vi "Contour.vi"(8 "error in (no error)":errorcluster, 10 "ContourParameter":T3={"ROI"={"Global Rectangle"=[], "Contours"=[]}, "Search Direction"=enum."Rect Left To Right", "Curve Extraction"={"Extraction Mode"=0, "Edge Threshold"=75, "Edge Filter Size"=1, "Min Length"=25, "Search Step Size"=15, "Max Endpoint Gap"=10, "Subpixel"=TRUE}, "Contour Selection"=enum."Closest To Search Start", "Curve Connection"=[]} {"Curve Connection"."Max" format="%.2f"; "Curve Connection"."Min" format="%.2f"; "Curve Connection"."Match Constraints" items=["Distance (pixel)", "Angle Difference (degrees)", "Connectivity Distance (pixel)", "Gradient Difference (degrees)"]; "Curve Extraction"."Extraction Mode" items=["Normal", "Uniform Regions"]; "Curve Extraction"."Edge Filter Size" items=["Fine", "Normal", "Contour Tracing"]; "Curve Extraction"."Max Endpoint Gap" min=0; "Curve Extraction"."Search Step Size" min=1 max=255 step=1; "Curve Extraction"."Min Length" min=0; "Curve Extraction"."Edge Threshold" min=1 max=350 step=1; "ROI"."Contours"."Type" items=["No Selection", "Point", "Line", "Rectangle", "Oval", "Polygon", "Free", "Annulus", "Unused2", "Unused3", "Broken Line", "Free Hand Line", "Rotated Rectangle"]}, 11 "Image In":T2) -> (0 "error out":errorcluster, 2 "ContourResult":T1, 3 "Image Out":T2)   [LabVIEW 2019]
uses:
  <vilib>/vision/Image Controls.llb/IMAQ Image.ctl
  Controls/Contour/Analysis_Contour_Parameter.ctl
  <vilib>/vision/Contour.llb/IMAQ Contour Curve Extraction.ctl
  <vilib>/vision/Contour.llb/IMAQ Connect Range Setting.ctl
  Controls/Contour/Analysis_Contour_Result.ctl
  <vilib>/vision/NI_Vision_Development_Module.lvlib
panel:
  # "Range"
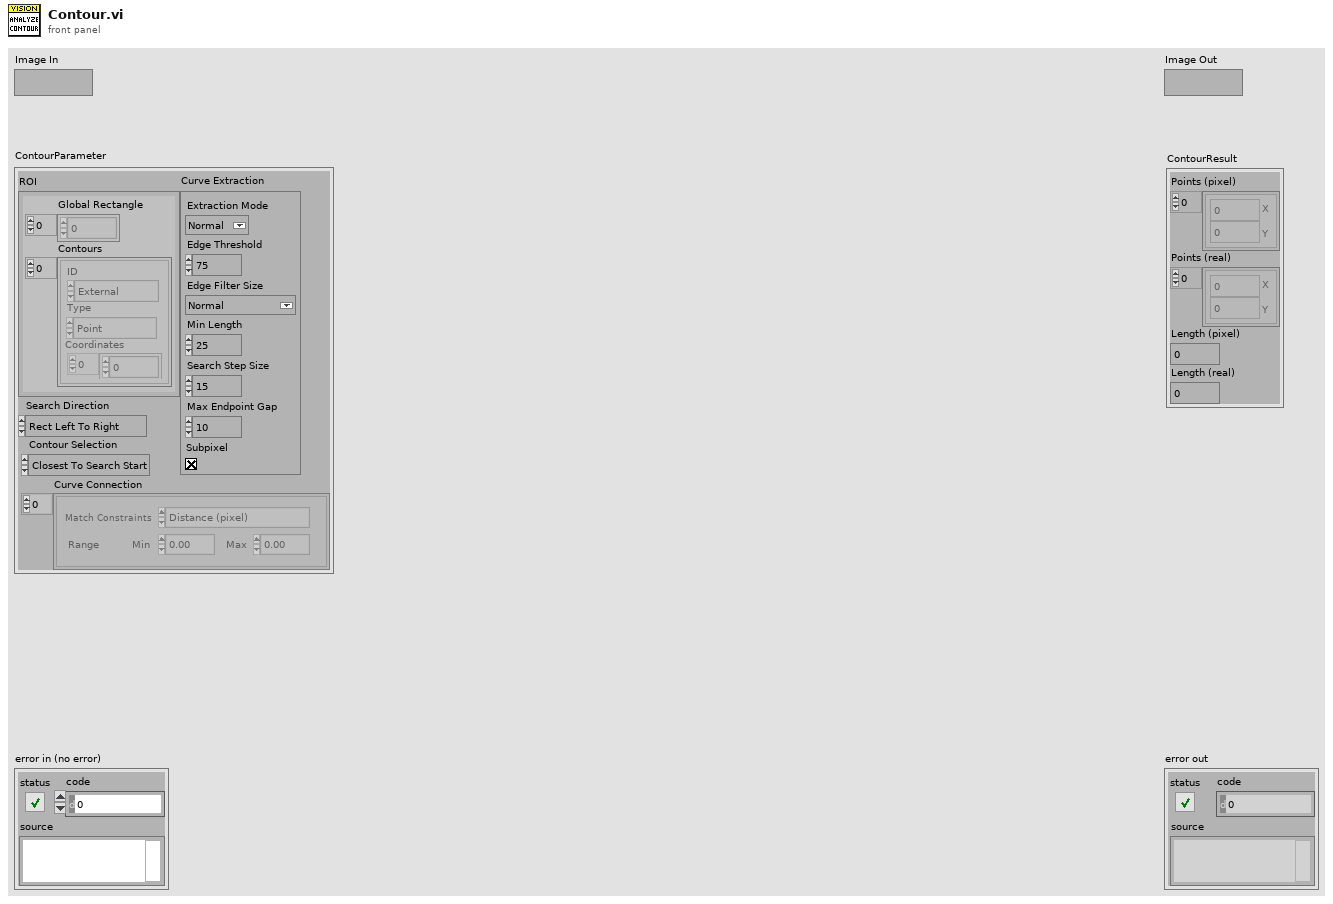
[diagram p1: front panel]
types:
  T1 = typedef "Analysis_Contour_Result.ctl" = cluster{"Points (pixel)":cluster{"X":dbl, "Y":dbl}[], "Points (real)":cluster{"X":dbl, "Y":dbl}[], "Length (pixel)":dbl, "Length (real)":dbl}
  T2 = typedef "IMAQ Image.ctl" = refnum<image>
  T3 = typedef "Analysis_Contour_Parameter.ctl" = cluster{"ROI":cluster{"Global Rectangle":i32[], "Contours":cluster{"ID":enum32{"External", "Internal"}, "Type":u32, "Coordinates":i32[]}[]}, "Search Direction":enum16{"Rect Left To Right", "Rect Right To Left", "Rect Top To Bottom", "Rect Bottom To Top", "Annulus Inner To Outer", "Annulus Outer To Inner", "Annulus Start Angle To End Angle", "Annulus End Angle To Start Angle"}, "Curve Extraction":T4, "Contour Selection":enum16{"Closest To Search Start", "Maximum Length", "Strongest Mean Gradient Change"}, "Curve Connection":T5[]}
  T4 = typedef "IMAQ Contour Curve Extraction.ctl" = cluster{"Extraction Mode":u32, "Edge Threshold":i32, "Edge Filter Size":u32, "Min Length":i32, "Search Step Size":i32, "Max Endpoint Gap":i32, "Subpixel":bool}
  T5 = typedef "IMAQ Connect Range Setting.ctl" = cluster{"Match Constraints":u32, "Min":dbl, "Max":dbl}
  T6 = cluster{"Overlay?":bool, "Color":u32, "Width":u32, "Maintain Width?":bool}
  T7 = cluster{"Global Rectangle":i32[], "Contours":cluster{"ID":enum32{"External", "Internal"}, "Type":u32, "Coordinates":i32[]}[]}
  T8 = enum16{"Rect Left To Right", "Rect Right To Left", "Rect Top To Bottom", "Rect Bottom To Top", "Annulus Inner To Outer", "Annulus Outer To Inner", "Annulus Start Angle To End Angle", "Annulus End Angle To Start Angle"}
  T9 = enum16{"Closest To Search Start", "Maximum Length", "Strongest Mean Gradient Change"}
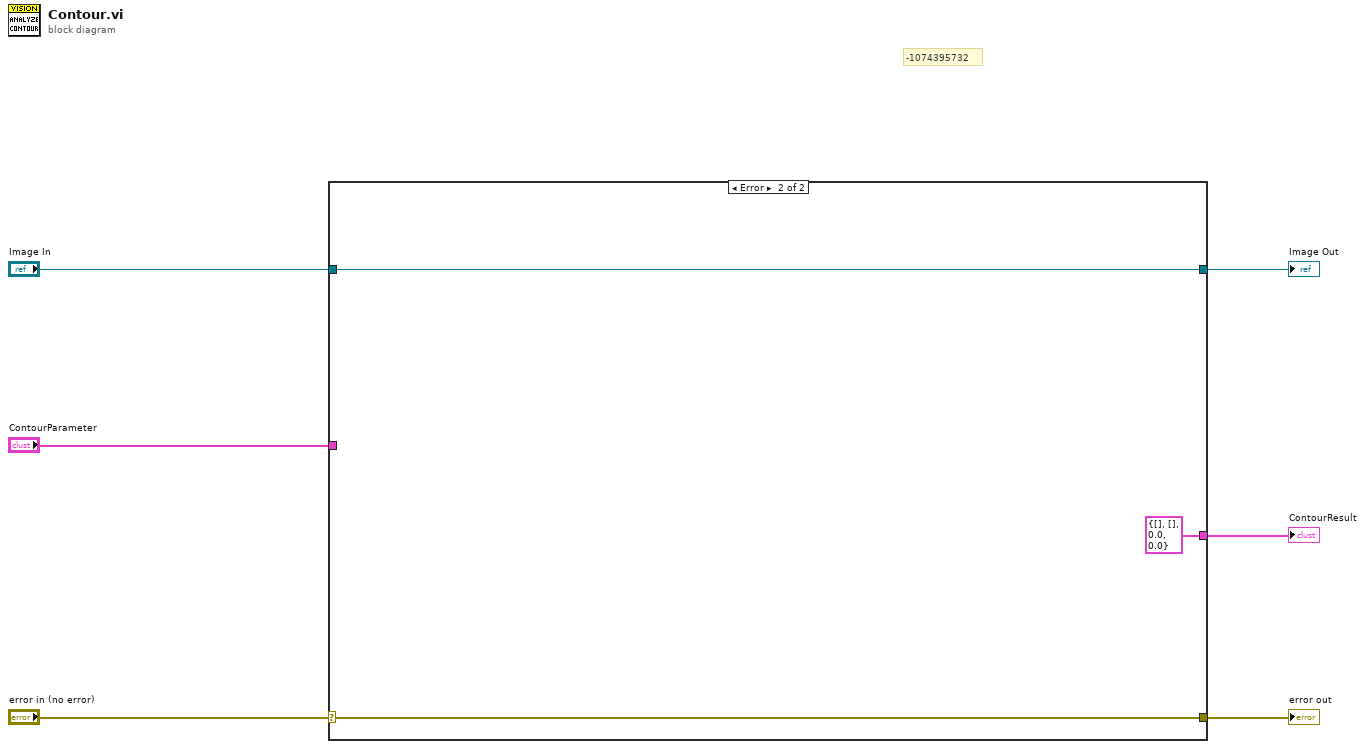
[diagram p0: block diagram]
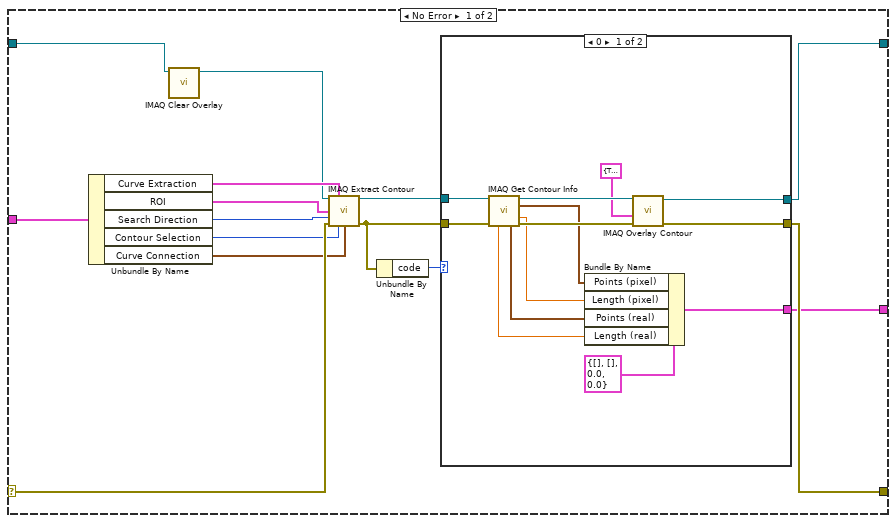
[diagram p2: hidden frame]
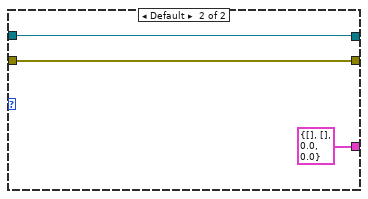
[diagram p3: hidden frame]
diagram:
  # "-1074395732"
  n1 = case shown="Error" "error in (no error)" {
    selector: "error in (no error)" -> [w20 w40]
    tunnel: [w12 w40] -> w5
    tunnel: "Image In" -> [w11 w39]
    tunnel: "ContourParameter" -> [w19 _]
    tunnel: [w13 w39] -> w2
    tunnel: [w7 T1 {"Points (pixel)"=[], "Points (real)"=[], "Length (pixel)"=0.0, "Length (real)"=0.0} ("ContourResult")] -> w1
    frame No Error {
      n2 = Unbundle By Name(w19) -> ("Curve Extraction"=w18:T4, "ROI"=w15:T7, "Search Direction"=w14:T8, "Contour Selection"=w16:T9, "Curve Connection"=w17:T5[])
      n3 = call "IMAQ Clear Overlay"("Image"=w11) -> ("Image Out"=w10:T2)  [unwired: 9 in, 1 out]
      n4 = call "IMAQ Extract Contour"("Source Image"=w10, "Curve Extraction"=w18, "ROI Descriptor"=w15, "Search Direction"=w14, "error in (no error)"=w20, "Contour Selection"=w16, "Curve Connection"=w17) -> ("Source Image Out"=w21:T2, "error out"=w9:errorcluster)  [unwired: 4 in, 3 out]
      n5 = Unbundle By Name(w9) -> ("code"=w8:i32)
      n6 = case shown="0" w8 {
        tunnel: w21 -> [w34 w37]
        tunnel: [w31 w37] -> w13
        tunnel: [w30 w36] -> w12
        tunnel: w9 -> [w28 w36]
        tunnel: [w22 T1 {"Points (pixel)"=[], "Points (real)"=[], "Length (pixel)"=0.0, "Length (real)"=0.0} ("ContourResult")] -> w7
        frame 0 {
          n7 = call "IMAQ Get Contour Info"("Contour Image"=w34, "error in (no error)"=w28) -> ("Contour Image Out (dup)"=w33:T2, "Points (pixel)"=w26:cluster{"X":dbl, "Y":dbl}[], "Length (pixel)"=w25:dbl, "Length (real)"=w23:dbl, "Points (real)"=w24:cluster{"X":dbl, "Y":dbl}[], "error out"=w32:errorcluster)  [unwired: 5 in, 3 out]
          n8 = Bundle By Name(cluster=T1 {"Points (pixel)"=[], "Points (real)"=[], "Length (pixel)"=0.0, "Length (real)"=0.0} ("ContourResult"), "Points (pixel)"=w26, "Length (pixel)"=w25, "Points (real)"=w24, "Length (real)"=w23) -> (w22:T1)
          n9 = call "IMAQ Overlay Contour"("error in (no error)"=w32, "Contour Points Settings"=T6 {"Overlay?"=TRUE, "Color"=16711680, "Width"=1, "Maintain Width?"=TRUE}, "Image"=w33) -> ("error out"=w30:errorcluster, "Image Out"=w31:T2)  [unwired: 7 in]
        }
        frame Default {
        }
      }
    }
    frame Error {
    }
  }
  "error out" <- w5
  "Image Out" <- w2
  "ContourResult" <- w1
